vi "9205_Read_Mod6.vi"(10 "error in":errorcluster) -> (2 "error out":errorcluster, 3 "data out":fxp<+/-,26,5>[](array[numeric]))   [LabVIEW 2015]
uses:
  <vilib>/rvi/eio/common/nirviEmuTemplateMethod_errors.vi
  <vilib>/eio/EIONode/EIONode.xnode
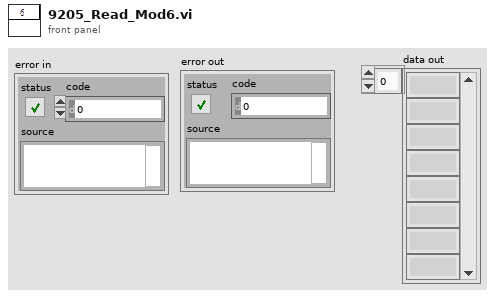
[diagram p1: front panel]
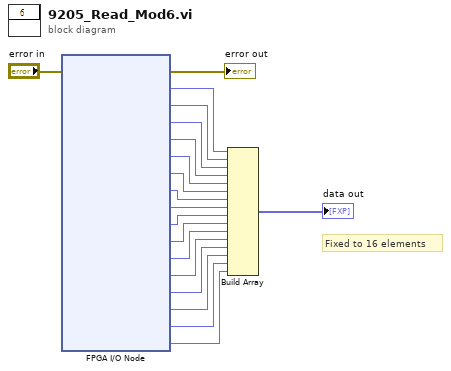
[diagram p0: block diagram]
diagram:
  # "Fixed to 16 elements"
  n1 = xnode "FPGA I/O Node"("error in"="error in") -> ("error out"=→"error out":errorcluster, "Mod6/AI0"=w19:fxp<+/-,26,5>, "Mod6/AI1"=w18:fxp<+/-,26,5>, "Mod6/AI2"=w17:fxp<+/-,26,5>, "Mod6/AI3"=w16:fxp<+/-,26,5>, "Mod6/AI4"=w15:fxp<+/-,26,5>, "Mod6/AI5"=w14:fxp<+/-,26,5>, "Mod6/AI6"=w13:fxp<+/-,26,5>, "Mod6/AI7"=w12:fxp<+/-,26,5>, "Mod6/AI16"=w11:fxp<+/-,26,5>, "Mod6/AI17"=w10:fxp<+/-,26,5>, "Mod6/AI18"=w9:fxp<+/-,26,5>, "Mod6/AI19"=w8:fxp<+/-,26,5>, "Mod6/AI20"=w7:fxp<+/-,26,5>, "Mod6/AI21"=w6:fxp<+/-,26,5>, "Mod6/AI22"=w5:fxp<+/-,26,5>, "Mod6/AI23"=w4:fxp<+/-,26,5>)  [unwired: 16 in, 16 out]
  n2 = Build Array(w19, w18, w17, w16, w15, w14, w13, w12, w11, w10, w9, w8, w7, w6, w5, w4) -> (→"data out":fxp<+/-,26,5>[])
